vi "Read VISA_Ref.vi"(8 "error in (no error)":errorcluster, 11 "RS232 In":refnum<class "RS232.lvclass">) -> (0 "error out":errorcluster, 2 "VISA_Ref":refnum<visa-resource-name>, 3 "RS232 Out":refnum<class "RS232.lvclass">)   [LabVIEW 2019, in "RS232.lvclass"]
uses:
  RS232.lvclass
  RS232.lvclass/RS232.ctl
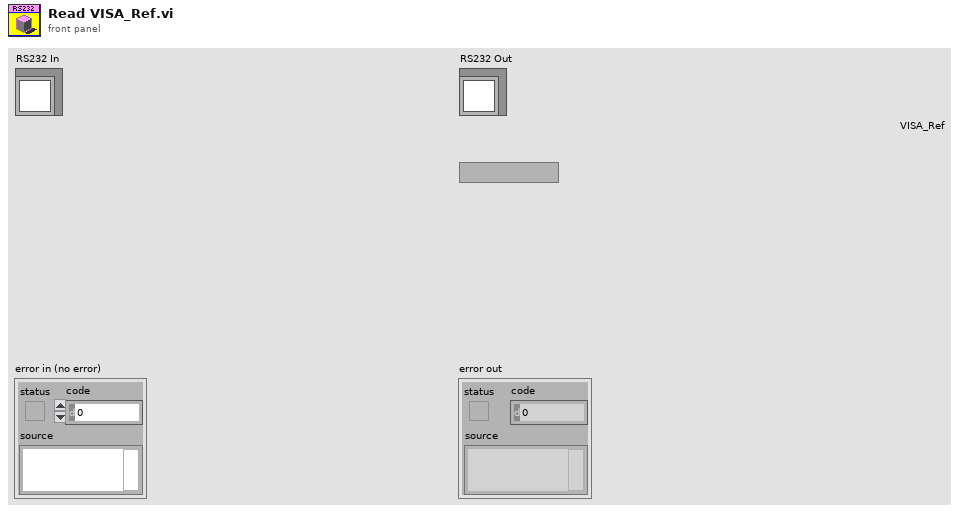
[diagram p1: front panel]
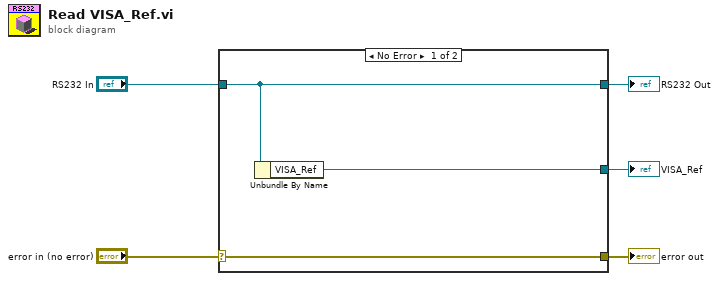
[diagram p0: block diagram]
diagram:
  n1 = case shown="No Error" "error in (no error)" {
    selector: "error in (no error)" -> [w8 w9]
    tunnel: [w8 w9] -> w4
    tunnel: [w7 w10] -> w2
    tunnel: "RS232 In" -> [w7 w10]
    tunnel: [w6 _] -> w1
    frame No Error {
      n2 = Unbundle By Name(w7) -> ("VISA_Ref"=w6:refnum<visa-resource-name>)
    }
    frame Error {
    }
  }
  "error out" <- w4
  "RS232 Out" <- w2
  "VISA_Ref" <- w1
